vi "configmgr-simpleread-test.vi"(8 "error in (no error)":errorcluster) -> (0 "error out":errorcluster)   [LabVIEW 2013]
uses:
  _test-support-SMOs/SMO.Configurable/Config--cluster.ctl
  src/SMO/Typedefs/SMOState --Enum.ctl
  <vilib>/addons/_JKI Toolkits/Caraya/classes/Test/Test.lvclass
  <vilib>/addons/_JKI Toolkits/Caraya/classes/Assert/Assert.lvclass
  _test-support-SMOs/SMO.Configurable/SMO.Configurable.lvclass
  src/SMO/SMO.lvclass
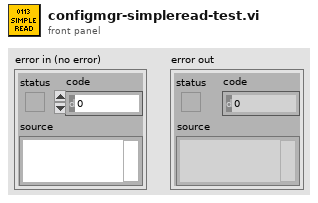
[diagram p1: front panel]
types:
  T1 = typedef "SMO.lvclass/SMOState --Enum.ctl" = enum16{"unknown", "Created", "Started", "Stopped"}
  T2 = typedef "SMO.Configurable.lvclass/Config--cluster.ctl" = cluster{"timeout":i32, "run":bool}
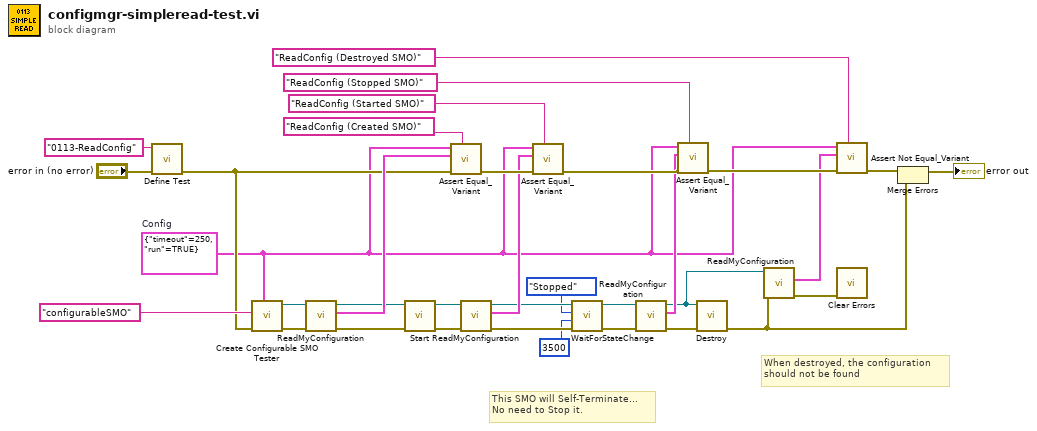
[diagram p0: block diagram]
diagram:
  w3 = T2 {"timeout"=250, "run"=TRUE}  # Config
  # "When destroyed, the configuration\nshould not be found"
  # "This SMO will Self-Terminate...\nNo need to Stop it."
  n1 = call <vilib>:"Define Test.vi"("error in (no error)"="error in (no error)", "Label (VI Title)"="0113-ReadConfig") -> ("error out"=w26:errorcluster)  [unwired: 9 in]
  n2 = call "Create Configurable SMO Tester.vi"("Config"=w3, "error in (no error)"=w26, "Subsystem Name (optional)"="configurableSMO") -> ("error out"=w28:errorcluster, "SMO.Configurable out"=w29:refnum<class "SMO.Configurable.lvclass">)  [unwired: 6 in, 1 out]
  n3 = call "ReadMyConfiguration.vi"("error in (no error)"=w28, "SMO.Configurable in"=w29) -> ("error out"=w25:errorcluster, "Config"=w27:T2, "SMO.Configurable out"=w24:refnum<class "SMO.Configurable.lvclass">)  [unwired: 7 in]
  n4 = call "Start.vi"("error in (no error)"=w25, "SMO"=w24) -> ("error out"=w21:errorcluster, "SMO out"=w23:refnum<class "SMO.Configurable.lvclass">)  [unwired: 8 in]
  n5 = call <vilib>:"Assert Equal_Variant.vi"("Label"="ReadConfig (Created SMO)" ("Label (VI Title)"), "error in (no error)"=w26, "Y"=w27, "X"=w3) -> ("error out"=w20:errorcluster)  [unwired: 7 in]
  n6 = call "ReadMyConfiguration.vi"("error in (no error)"=w21, "SMO.Configurable in"=w23) -> ("error out"=w12:errorcluster, "Config"=w19:T2, "SMO.Configurable out"=w14:refnum<class "SMO.Configurable.lvclass">)  [unwired: 7 in]
  n7 = call <vilib>:"Assert Equal_Variant.vi"("Label"="ReadConfig (Started SMO)" ("Label (VI Title)"), "error in (no error)"=w20, "Y"=w19, "X"=w3) -> ("error out"=w18:errorcluster)  [unwired: 7 in]
  n8 = call "WaitForStateChange.vi"("error in (no error)"=w12, "timeout in ms (-1)"=3500, "State (unknown: Any state change)"=SMOState_--Enum."Stopped", "SMO in"=w14) -> ("error out"=w11:errorcluster, "SMO out"=w13:refnum<class "SMO.Configurable.lvclass">)  [unwired: 5 in, 1 out]
  n9 = call "ReadMyConfiguration.vi"("error in (no error)"=w11, "SMO.Configurable in"=w13) -> ("error out"=w22:errorcluster, "Config"=w15:T2, "SMO.Configurable out"=w8:refnum<class "SMO.Configurable.lvclass">)  [unwired: 7 in]
  n10 = call <vilib>:"Assert Equal_Variant.vi"("Label"="ReadConfig (Stopped SMO)" ("Label (VI Title)"), "error in (no error)"=w18, "Y"=w15, "X"=w3) -> ("error out"=w5:errorcluster)  [unwired: 7 in]
  n11 = call "Destroy.vi"("error in (no error)"=w22, "SMO"=w8) -> ("error out"=w7:errorcluster)  [unwired: 9 in]
  n12 = call "ReadMyConfiguration.vi"("error in (no error)"=w7, "SMO.Configurable in"=w8) -> ("error out"=w1:errorcluster, "Config"=w2:T2)  [unwired: 7 in, 1 out]
  n13 = call <vilib>:"Assert Not Equal_Variant.vi"("Label"="ReadConfig (Destroyed SMO)" ("Label (VI Title)"), "error in (no error)"=w5, "Y"=w2, "X"=w3) -> ("error out"=w6:errorcluster)  [unwired: 7 in]
  n14 = call <vilib>:"Clear Errors.vi"("error in (no error)"=w1) -> ()  [unwired: 6 in, 1 out]
  n15 = Merge Errors(w6, w7) -> (→"error out":errorcluster)
